vi "node.vi"() -> ()   [LabVIEW 2013]
panel:
  in  "Write":bool
  in  "data in":string
  in  "stop":bool
  out "data out":string
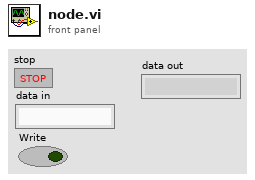
[diagram p1: front panel]
types:
  T1 = enum16{"Standard", "Buffered", "CRLF", "Immediate"}
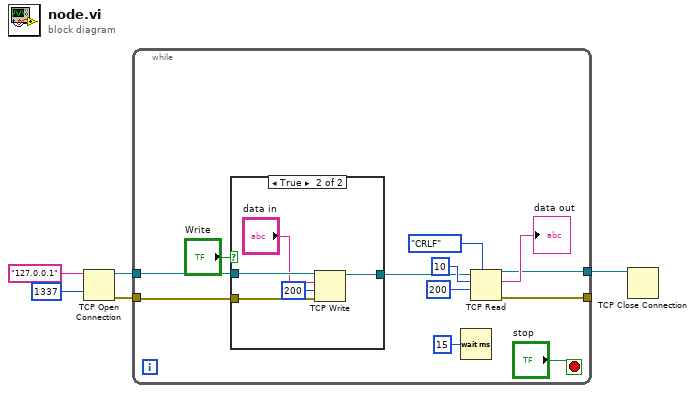
[diagram p0: block diagram]
diagram:
  n1 = TCP Open Connection(address="127.0.0.1", remote port or service name=u16 1337) -> (connection ID=w3:refnum<k5>, error out=w2:errorcluster)  [unwired: 3 in]
  n2 = while {
    tunnel: w3 -> [w9]
    tunnel: w2 -> [w7]
    tunnel: [w12] -> _
    tunnel: [w11] -> w1
    stop <- "stop" stop-if-true
    n3 = case shown="True" "Write" {
      tunnel: w9 -> [w18 w23]
      tunnel: [w18 w22] -> w8
      tunnel: w7 -> [_ w21]
      frame False {
      }
      frame True {
        n4 = TCP Write(connection ID=w23, data in="data in", error in (no error)=w21, 9:200 ("timeout ms (25000)")) -> (connection ID out=w22:refnum<k5>)  [unwired: 2 out]
      }
    }
    n5 = Wait (ms)(milliseconds to wait=u32 15) -> ()  [unwired: 1 out]
    n6 = TCP Read(connection ID=w8, bytes to read=10, 7:T1."CRLF" ("mode (standard)"), 9:200 ("timeout ms (25000)")) -> (connection ID out=w11:refnum<k5>, data out=→"data out":string, error out=w12:errorcluster)  [unwired: 1 in]
  }
  n7 = TCP Close Connection(connection ID=w1) -> ()  [unwired: 2 in, 2 out]
